vi "Halvorsen_1D_New.vi"(11 "Initial Conditions":ext[](array[numeric])=[0.1, 0.1, 0.1]) -> ()   [LabVIEW 2016]
panel:
  in  "Tab Control":enum32{"Mode Analysis", "Time Domain"}(tab)
  out "Mode Analysis":cluster{ext[], dbl[]}[](graph)=[{[1.4, 1.4050000000000000001, 1.4100000000000000002, 1.4150000000000000003, 1.4200000000000000004, 1.4250000000000000005, 1.4300000000000000006, 1.4350000000000000007, 1.4400000000000000008, 1.4450000000000000009, 1.450000000000000001, 1.4550000000000000011, 1.4600000000000000012, 1.4650000000000000013, 1.4700000000000000014, 1.4750000000000000015, 1.48000000000000000164, 1.48500000000000000175, 1.49000000000000000185, 1.49500000000000000196, 1.5000000000000000021, 1.5050000000000000022, 1.5100000000000000023, 1.5150000000000000024, 1.5200000000000000025, 1.5250000000000000026, 1.5300000000000000027, 1.5350000000000000028, 1.5400000000000000029, 1.545000000000000003, 1.5500000000000000031, 1.5550000000000000032, 1.5600000000000000033, 1.5650000000000000034, 1.5700000000000000035, 1.5750000000000000036, 1.5800000000000000037, 1.5850000000000000038, 1.5900000000000000039, 1.595000000000000004, 1.6000000000000000041, 1.60500000000000000425, 1.61000000000000000435, 1.61500000000000000445, 1.6200000000000000046, 1.6250000000000000047, 1.6300000000000000048, 1.6350000000000000049, 1.640000000000000005, 1.6450000000000000051, 1.6500000000000000052, 1.6550000000000000053, 1.6600000000000000054, 1.6650000000000000055, 1.6700000000000000056, 1.6750000000000000057, 1.6800000000000000058, 1.6850000000000000059, 1.690000000000000006, 1.6950000000000000061, 1.7000000000000000062, 1.7050000000000000063, 1.7100000000000000064, 1.7150000000000000065, 1.7200000000000000066, 1.7250000000000000067, 1.73000000000000000685, 1.73500000000000000695, 1.7400000000000000071, 1.7450000000000000072, 1.7500000000000000073, 1.7550000000000000074, 1.7600000000000000075, 1.7650000000000000076, 1.7700000000000000077, 1.7750000000000000078, 1.7800000000000000079, 1.785000000000000008, 1.7900000000000000081, 1.7950000000000000082, 1.8000000000000000083, 1.8050000000000000084, 1.8100000000000000085, 1.8150000000000000086, 1.8200000000000000087, 1.8250000000000000088, 1.8300000000000000089, 1.835000000000000009, 1.8400000000000000091, 1.8450000000000000092, 1.8500000000000000093, 1.8550000000000000094, 1.8600000000000000096, 1.8650000000000000097, 1.8700000000000000098, 1.8750000000000000099, 1.88000000000000001, 1.8850000000000000101, 1.8900000000000000102, 1.8950000000000000103, 1.9000000000000000104, 1.9050000000000000105, 1.9100000000000000106, 1.9150000000000000107, 1.9200000000000000108, 1.9250000000000000109, 1.930000000000000011, 1.9350000000000000111, 1.9400000000000000112, 1.9450000000000000113, 1.9500000000000000114, 1.9550000000000000115, 1.9600000000000000116, 1.9650000000000000117, 1.9700000000000000118, 1.975000000000000012, 1.980000000000000012, 1.9850000000000000122, 1.9900000000000000123, 1.9950000000000000124], [1.0, 32.0, 32.0, 32.0, 32.0, 32.0, 32.0, 32.0, 32.0, 32.0, 32.0, 32.0, 32.0, 32.0, 32.0, 32.0, 32.0, 32.0, 32.0, 32.0, 32.0, 32.0, 32.0, 32.0, 32.0, 32.0, 32.0, 32.0, 32.0, 32.0, 32.0, 32.0, 2.0, 32.0, 32.0, 32.0, 32.0, 32.0, 32.0, 32.0, 32.0, 32.0, 32.0, 32.0, 32.0, 32.0, 32.0, 32.0, 32.0, 32.0, 32.0, 32.0, 32.0, 32.0, 32.0, 32.0, 10.0, 32.0, 32.0, 32.0, 32.0, 32.0, 32.0, 32.0, 32.0, 32.0, 32.0, 32.0, 8.0, 4.0, 4.0, 6.0, 13.0, 13.0, 3.0, 14.0, 8.0, 5.0, 3.0, 2.0, 2.0, 2.0, 2.0, 2.0, 2.0, 2.0, 2.0, 2.0, 2.0, 2.0, 2.0, 2.0, 2.0, 2.0, 2.0, 2.0, 2.0, 2.0, 2.0, 2.0, 2.0, 5.0, 2.0, 2.0, 2.0, 2.0, 2.0, 3.0, 2.0, 2.0, 2.0, 2.0, 2.0, 2.0, 2.0, 2.0, 2.0, 2.0, 2.0, 2.0]}, {[1.4, 1.4050000000000000001, 1.4100000000000000002, 1.4150000000000000003, 1.4200000000000000004, 1.4250000000000000005, 1.4300000000000000006, 1.4350000000000000007, 1.4400000000000000008, 1.4450000000000000009, 1.450000000000000001, 1.4550000000000000011, 1.4600000000000000012, 1.4650000000000000013, 1.4700000000000000014, 1.4750000000000000015, 1.48000000000000000164, 1.48500000000000000175, 1.49000000000000000185, 1.49500000000000000196, 1.5000000000000000021, 1.5050000000000000022, 1.5100000000000000023, 1.5150000000000000024, 1.5200000000000000025, 1.5250000000000000026, 1.5300000000000000027, 1.5350000000000000028, 1.5400000000000000029, 1.545000000000000003, 1.5500000000000000031, 1.5550000000000000032, 1.5600000000000000033, 1.5650000000000000034, 1.5700000000000000035, 1.5750000000000000036, 1.5800000000000000037, 1.5850000000000000038, 1.5900000000000000039, 1.595000000000000004, 1.6000000000000000041, 1.60500000000000000425, 1.61000000000000000435, 1.61500000000000000445, 1.6200000000000000046, 1.6250000000000000047, 1.6300000000000000048, 1.6350000000000000049, 1.640000000000000005, 1.6450000000000000051, 1.6500000000000000052, 1.6550000000000000053, 1.6600000000000000054, 1.6650000000000000055, 1.6700000000000000056, 1.6750000000000000057, 1.6800000000000000058, 1.6850000000000000059, 1.690000000000000006, 1.6950000000000000061, 1.7000000000000000062, 1.7050000000000000063, 1.7100000000000000064, 1.7150000000000000065, 1.7200000000000000066, 1.7250000000000000067, 1.73000000000000000685, 1.73500000000000000695, 1.7400000000000000071, 1.7450000000000000072, 1.7500000000000000073, 1.7550000000000000074, 1.7600000000000000075, 1.7650000000000000076, 1.7700000000000000077, 1.7750000000000000078, 1.7800000000000000079, 1.785000000000000008, 1.7900000000000000081, 1.7950000000000000082, 1.8000000000000000083, 1.8050000000000000084, 1.8100000000000000085, 1.8150000000000000086, 1.8200000000000000087, 1.8250000000000000088, 1.8300000000000000089, 1.835000000000000009, 1.8400000000000000091, 1.8450000000000000092, 1.8500000000000000093, 1.8550000000000000094, 1.8600000000000000096, 1.8650000000000000097, 1.8700000000000000098, 1.8750000000000000099, 1.88000000000000001, 1.8850000000000000101, 1.8900000000000000102, 1.8950000000000000103, 1.9000000000000000104, 1.9050000000000000105, 1.9100000000000000106, 1.9150000000000000107, 1.9200000000000000108, 1.9250000000000000109, 1.930000000000000011, 1.9350000000000000111, 1.9400000000000000112, 1.9450000000000000113, 1.9500000000000000114, 1.9550000000000000115, 1.9600000000000000116, 1.9650000000000000117, 1.9700000000000000118, 1.975000000000000012, 1.980000000000000012, 1.9850000000000000122, 1.9900000000000000123, 1.9950000000000000124], [0.0, 32.0, 32.0, 32.0, 32.0, 32.0, 32.0, 32.0, 32.0, 32.0, 32.0, 32.0, 32.0, 32.0, 32.0, 32.0, 32.0, 32.0, 32.0, 32.0, 32.0, 32.0, 32.0, 32.0, 32.0, 32.0, 32.0, 32.0, 32.0, 32.0, 32.0, 21.0, 2.0, 32.0, 32.0, 32.0, 32.0, 32.0, 32.0, 32.0, 32.0, 32.0, 32.0, 32.0, 32.0, 32.0, 32.0, 32.0, 32.0, 32.0, 32.0, 32.0, 32.0, 32.0, 32.0, 32.0, 6.0, 32.0, 32.0, 32.0, 32.0, 32.0, 32.0, 32.0, 32.0, 32.0, 32.0, 32.0, 7.0, 4.0, 4.0, 5.0, 12.0, 8.0, 3.0, 3.0, 3.0, 2.0, 2.0, 2.0, 2.0, 2.0, 2.0, 2.0, 2.0, 2.0, 2.0, 2.0, 2.0, 2.0, 2.0, 2.0, 2.0, 2.0, 2.0, 2.0, 2.0, 2.0, 2.0, 2.0, 2.0, 6.0, 3.0, 2.0, 2.0, 2.0, 2.0, 3.0, 2.0, 2.0, 2.0, 2.0, 2.0, 2.0, 2.0, 2.0, 2.0, 2.0, 2.0, 2.0]}]
  out "Waveform Graph":ext[][](graph)
  out "Bifurcation Diagram":cluster{ext[], ext[]}(graph)
  in  "Parameter Index":i32=1
  in  "Final Parameter Value":dbl=2.0
  in  "Param_Inc":dbl[](array[numeric])=[0.0, 0.005, 0.0]
  in  "Initial_Parameter_Vector":ext[](array[numeric])=[1.4, 1.4, 1.4]
  out "Current_Param":ext[](array[numeric])=[1.4, 2.0000000000000000126, 1.4]
  in  "Variable":u16(ring) items=["x", "y", "z"]
  in  "Время, с":ext=500.0
  in  "Hmin":ext=0.00099999999999999999996
  in  "Hmax":ext=1.0
  in  "tolerance":ext=1e-11
  in  "Шаг h, с":ext=0.01
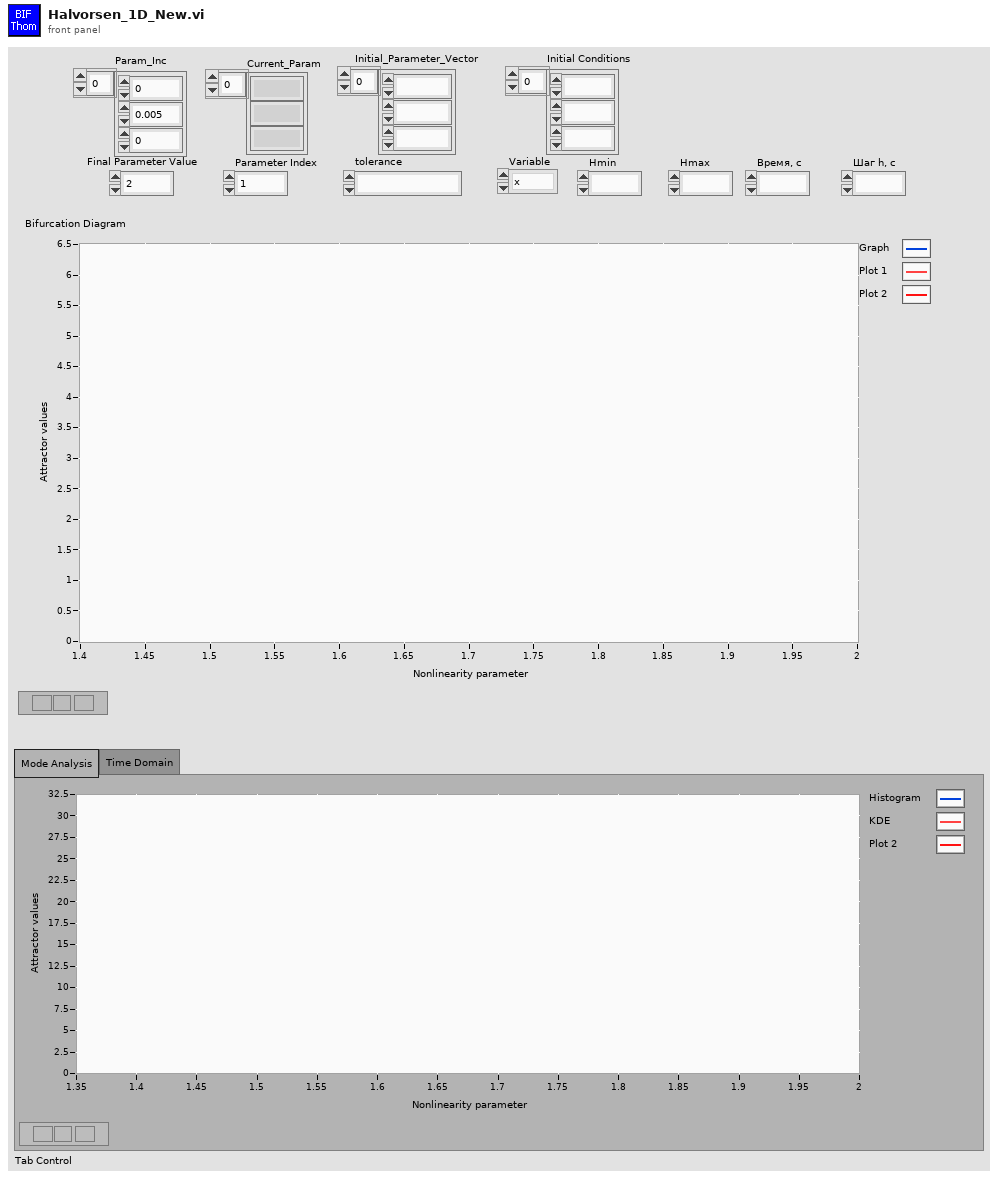
[diagram p1: front panel]
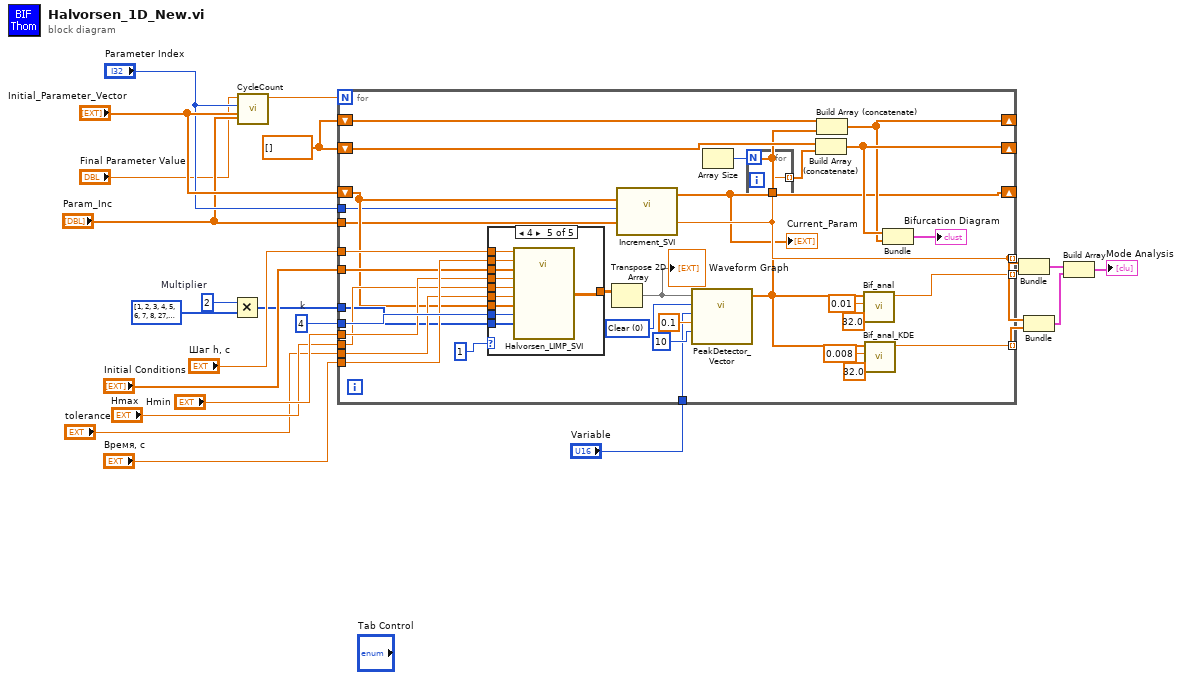
[diagram p0: block diagram]
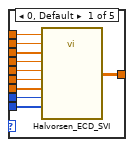
[diagram p2: hidden frame]
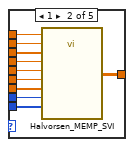
[diagram p3: hidden frame]
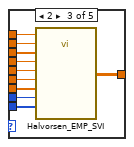
[diagram p4: hidden frame]
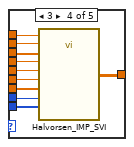
[diagram p5: hidden frame]
diagram:
  w7 = ext[] []
  w9 = 4  # k
  w12 = 2  # Multiplier
  n1 = Multiply(x=w12, y=i32[] [1, 2, 3, 4, 5, 6, 7, 8, 27, 30, 33] ("n")) -> (x*y=w10:i32[])
  n2 = call "CycleCount.vi"("Increment_Vector"="Param_Inc", "Parameter_Vector"="Initial_Parameter_Vector", "Parameter Number"="Parameter Index", "Final_Parameter_Value"="Final Parameter Value") -> ("Cycle Count"=w8:ext)  [unwired: 5 in, 2 out]
  n3 = for {
    N: w8 -> [_]
    tunnel: w9 -> [w57]
    tunnel: "Шаг h, с" -> [w46]
    tunnel: "Время, с" -> [w56]
    tunnel: "tolerance" -> [w55]
    tunnel: "Hmin" -> [w54]
    tunnel: "Hmax" -> [w53]
    tunnel: w10 -> [w52]
    tunnel: "Initial Conditions" -> [w51]
    shift-right: [w24] -> _
    shift-left: "Initial_Parameter_Vector" -> [w45]
    tunnel: "Parameter Index" -> [w44]
    tunnel: "Param_Inc" -> [w43]
    tunnel: [w42] -> w6 mode=indexing
    tunnel: "Variable" -> [w41]
    shift-right: [w33] -> _
    shift-left: w7 -> [w38]
    shift-right: [w34] -> _
    shift-left: w7 -> [w37]
    tunnel: [w32] -> w3 mode=indexing
    tunnel: [w26] -> w2 mode=indexing
    w49 = u16 0 items=["Clear", "Absolute", "Positive"] ("Signal Mode")
    n4 = case shown="4" 1 {
      tunnel: w57 -> [w68 w78 w80 w90 w101]
      tunnel: w56 -> [w67 w77 w86 w96 w107]
      tunnel: w55 -> [w66 w76 w82 w92 w103]
      tunnel: w54 -> [w65 w75 w84 w94 w105]
      tunnel: w53 -> [w64 w74 w83 w93 w104]
      tunnel: w52 -> [w63 w73 w79 w89 w100]
      tunnel: w51 -> [w62 w72 w85 w95 w106]
      tunnel: [w61 w71 w88 w98 w99] -> w50
      tunnel: w46 -> [w60 w70 w87 w97 w108]
      tunnel: w45 -> [w59 w69 w81 w91 w102]
      frame 0, Default {
        n5 = call "Halvorsen_ECD_SVI.vi"("Шаг h, с"=w60, "n"=w63, "k"=w68, "Parameter_Vector"=w59, "Время, с"=w67, "Initial Conditions"=w62, "Hmin"=w65, "Hmax"=w64, "tolerance"=w66) -> ("Solution"=w61:ext[][])  [unwired: 6 in]
      }
      frame 1 {
        n6 = call "Halvorsen_MEMP_SVI.vi"("Шаг h, с"=w70, "n"=w73, "k"=w78, "Parameter_Vector"=w69, "Время, с"=w77, "Initial Conditions"=w72, "Hmin"=w75, "Hmax"=w74, "tolerance"=w76) -> ("Solution"=w71:ext[][])  [unwired: 6 in]
      }
      frame 2 {
        n7 = call "Halvorsen_EMP_SVI.vi"("Шаг h, с"=w87, "n"=w79, "k"=w80, "Parameter_Vector"=w81, "Время, с"=w86, "Initial Conditions"=w85, "Hmin"=w84, "Hmax"=w83, "tolerance"=w82) -> ("Solution"=w88:ext[][])  [unwired: 6 in]
      }
      frame 3 {
        n8 = call "Halvorsen_IMP_SVI.vi"("Шаг h, с"=w97, "n"=w89, "k"=w90, "Parameter_Vector"=w91, "Время, с"=w96, "Initial Conditions"=w95, "Hmin"=w94, "Hmax"=w93, "tolerance"=w92) -> ("Solution"=w98:ext[][])  [unwired: 6 in]
      }
      frame 4 {
        n9 = call "Halvorsen_LIMP_SVI.vi"("Шаг h, с"=w108, "n"=w100, "k"=w101, "Parameter_Vector"=w102, "Время, с"=w107, "Initial Conditions"=w106, "Hmin"=w105, "Hmax"=w104, "tolerance"=w103) -> ("Solution"=w99:ext[][])  [unwired: 6 in]
      }
    }
    n10 = Transpose 2D Array(2D array=w50) -> (transposed array=w25:ext[][])
    "Waveform Graph" <- w25
    n11 = call "Increment_SVI.vi"("Increment_Vector"=w43, "Param_Index"=w44, "Parameter_Vector"=w45) -> ("Current_Parameter"=w32:ext, "Parameters_Out"=w24:ext[])  [unwired: 7 in]
    "Current_Param" <- w24
    n12 = call "PeakDetector_Vector.vi"("threshold"=0.1, "FWD cut length"=10, "Variable_Num"=w41, "Signal Mode"=w49, "Input signal"=w25) -> ("Out signal"=w27:dbl[])  [unwired: 5 in, 1 out]
    n13 = Array Size(array=w27) -> (size(s)=w39:i32)
    n14 = for {
      N: w39 -> [_]
      tunnel: [w58] -> w35 mode=indexing
      tunnel: w32 -> [w58]
    }
    n15 = Build Array (concatenate)(w37, w35) -> (w34:ext[])
    n16 = Build Array (concatenate)(w38, w27) -> (w33:ext[])
    n17 = call "Bif_anal.vi"("n"=32.0, "Treshold"=0.01, "X"=w27) -> ("Y"=w42:dbl)  [unwired: 7 in, 1 out]
    n18 = call "Bif_anal_KDE.vi"("n"=32.0, "Manual h"=0.008 ("Treshold"), "X"=w27) -> ("Y"=w26:dbl)  [unwired: 7 in, 1 out]
    n19 = Bundle(w34, w33) -> (→"Bifurcation Diagram":cluster{ext[], ext[]})  [unwired: 1 in]
  }
  n20 = Bundle(w3, w6) -> (w5:cluster{ext[], dbl[]})  [unwired: 1 in]
  n21 = Bundle(w3, w2) -> (w1:cluster{ext[], dbl[]})  [unwired: 1 in]
  n22 = Build Array(w5, w1) -> (→"Mode Analysis":cluster{ext[], dbl[]}[])
